vi "Ramp Pattern by Delta.vi"(9 "start":dbl, 10 "end":dbl=1.0, 11 "delta":dbl) -> (0 "error":i32, 2 "samples":i32, 3 "Ramp Pattern":dbl[](array[numeric]))   [LabVIEW 2017, in "NI_AALBase.lvlib"]
doc: "Generates an array containing a ramp pattern. You must manually select the polymorphic instance you want to use."
uses:
  <vilib>/Analysis/NI_AALBase.lvlib
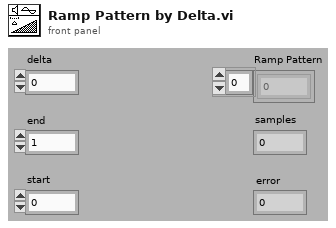
[diagram p1: front panel]
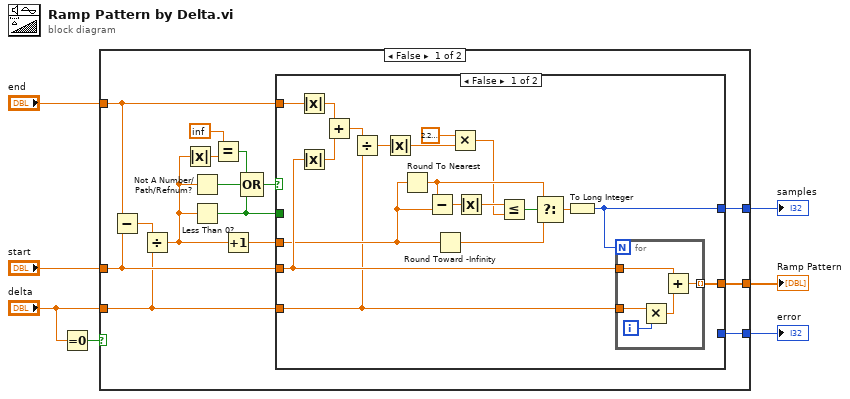
[diagram p0: block diagram]
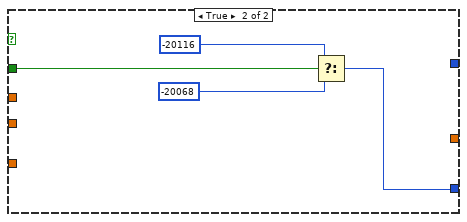
[diagram p2: hidden frame]
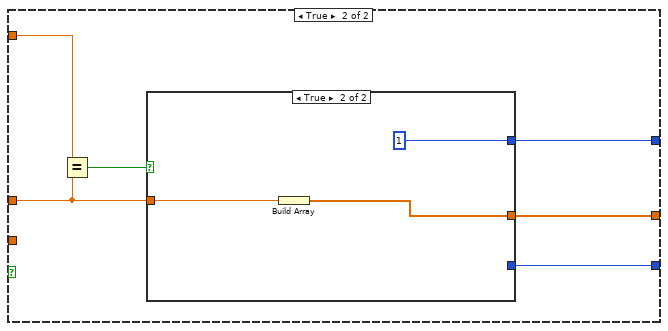
[diagram p3: hidden frame]
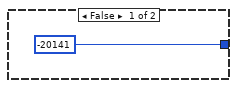
[diagram p4: hidden frame]
diagram:
  n1 = Equal To 0?(x="delta") -> (x = 0?=w2:bool)
  n2 = case shown="False" w2 {
    tunnel: "end" -> [w10 w55]
    tunnel: "start" -> [w21 w53]
    tunnel: [w20 w52] -> w5
    tunnel: [w19 w51] -> w4
    tunnel: "delta" -> [w18 _]
    tunnel: [w12 w56] -> w1
    frame False {
      n3 = Subtract(x=w10, y=w21) -> (x-y=w22:dbl)
      n4 = Divide(x=w22, y=w18) -> (x/y=w9:dbl)
      n5 = Absolute Value(x=w9) -> (abs(x)=w16:dbl)
      n6 = Not A Number/Path/Refnum?(number/path/refnum=w9) -> (NaN/Path/Refnum?=w14:bool)
      n7 = Less Than 0?(x=w9) -> (x < 0?=w11:bool)
      n8 = Equal?(x=inf, y=w16) -> (x = y?=w15:bool)
      n9 = Increment(x=w9) -> (x+1=w8:dbl)
      n10 = Compound Arithmetic op=OR(w15, w14, w11) -> (w13:bool)
      n11 = case shown="False" w13 {
        tunnel: w21 -> [w35 _]
        tunnel: [w41 _] -> w20
        tunnel: [w37 _] -> w19
        tunnel: w18 -> [w30 _]
        tunnel: [_ w48] -> w12
        tunnel: w11 -> [_ w50]
        tunnel: w10 -> [w36 _]
        tunnel: w8 -> [w32 _]
        frame False {
          n12 = Absolute Value(x=w36) -> (abs(x)=w34:dbl)
          n13 = Absolute Value(x=w35) -> (abs(x)=w33:dbl)
          n14 = Add(x=w34, y=w33) -> (x+y=w31:dbl)
          n15 = Divide(x=w31, y=w30) -> (x/y=w29:dbl)
          n16 = Absolute Value(x=w29) -> (abs(x)=w24:dbl)
          n17 = Round To Nearest(number=w32) -> (nearest integer value=w39:dbl)
          n18 = Subtract(x=w39, y=w32) -> (x-y=w28:dbl)
          n19 = Round Toward -Infinity(1:w32) -> (0:w40:dbl)
          n20 = Multiply(x=2.220446049250313e-16, y=w24) -> (x*y=w23:dbl)
          n21 = Absolute Value(x=w28) -> (abs(x)=w27:dbl)
          n22 = Less Or Equal?(x=w27, y=w23) -> (x <= y?=w26:bool)
          n23 = Select(t=w39, s=w26, f=w40) -> (s? t:f=w38:dbl)
          n24 = To Long Integer(number=w38) -> (32bit integer=w37:i32)
          n25 = for {
            N: w37 -> [_]
            tunnel: w30 -> [w45]
            tunnel: w35 -> [w43]
            tunnel: [w42] -> w41 mode=indexing
            i -> [w46]
            n26 = Multiply(x=w45, y=w46) -> (x*y=w44:dbl)
            n27 = Add(x=w43, y=w44) -> (x+y=w42:dbl)
          }
        }
        frame True {
          n28 = Select(t=-20116, s=w50, f=-20068) -> (s? t:f=w48:i32)
        }
      }
    }
    frame True {
      n29 = Equal?(x=w55, y=w53) -> (x = y?=w54:bool)
      n30 = case shown="True" w54 {
        tunnel: [-20141 _] -> w56
        tunnel: w53 -> [_ w60]
        tunnel: [_ w59] -> w52
        tunnel: [_ 1] -> w51
        frame False {
        }
        frame True {
          n31 = Build Array(w60) -> (w59:dbl[])
        }
      }
    }
  }
  "error" <- w1
  "Ramp Pattern" <- w5
  "samples" <- w4
